vi "Start High-Speed Data Communication.vi"(0 "Device ID":i32, 1 "Max Buffer Size":u32, 7 "Ethernet Config":T1={"IP Address"=[192, 168, 0, 1], "Port No"=24692}, 9 "Start Req":T2={"High-Speed Comm Start Pos"=0, "Read Profile Cnt"=0, "High-Speed Receive Ratio"=16} {"High-Speed Receive Ratio" items=["LOWEST"=0, "LOW"=16, "MIDDLE"=17, "HIGH"=18, "HIGHEST"=32]; "High-Speed Comm Start Pos" items=["SEND COMPLETE POS", "OLDEST", "NEXT"]}, 11 "error in (no error)":errorcluster {"code" format="%.0x"}) -> (4 "Device ID out":i32, 15 "error out":errorcluster {"code" format="%.0x"})   [LabVIEW 2010, in "KEYENCE LJ-X8000A.lvlib"]
doc: "High-speed communication with the controller is established to start."
uses:
  KEYENCE LJ-X8000A.lvlib
  Clusters/Ethernet Config.ctl
  Clusters/High-Speed Comm Start Req.ctl
  Constants/High-Speed Comm Start Pos.ctl
  Constants/High-Speed Receive Ratio.ctl
panel:
  # "(c) 2019 KEYENCE CORPORATION.  ALL RIGHTS RESERVED."
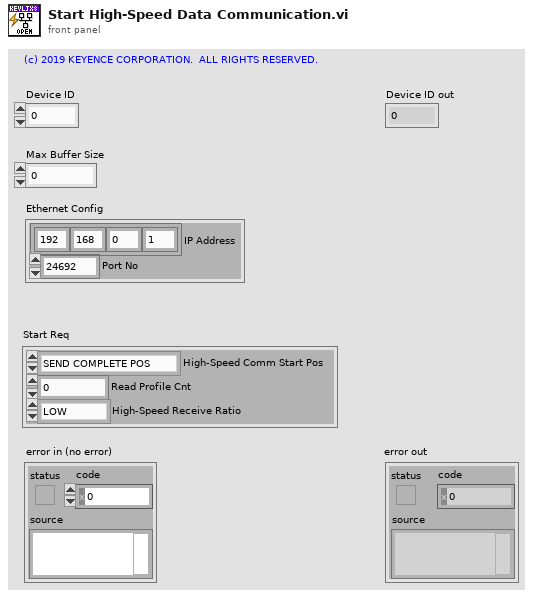
[diagram p1: front panel]
types:
  T1 = typedef "KEYENCE LJ-X8000A.lvlib/Ethernet Config.ctl" = cluster{"IP Address":u8[], "Port No":u16}
  T2 = typedef "KEYENCE LJ-X8000A.lvlib/High-Speed Comm Start Req.ctl" = cluster{"High-Speed Comm Start Pos":T3, "Read Profile Cnt":u32, "High-Speed Receive Ratio":T4}
  T3 = typedef "KEYENCE LJ-X8000A.lvlib/High-Speed Comm Start Pos.ctl" = u8
  T4 = typedef "KEYENCE LJ-X8000A.lvlib/High-Speed Receive Ratio.ctl" = u8
  T5 = cluster{"High-Speed Comm Start Pos":T3, "reserved":u8, "reserved":u8, "reserved":u8}
  T6 = cluster{"IP Address[0]":u8, "IP Address[1]":u8, "IP Address[2]":u8, "IP Address[3]":u8}
  T7 = cluster{"IP Address":cluster{"IP Address[0]":u8, "IP Address[1]":u8, "IP Address[2]":u8, "IP Address[3]":u8}, "Port No":u16, "reserved":u8, "reserved":u8}
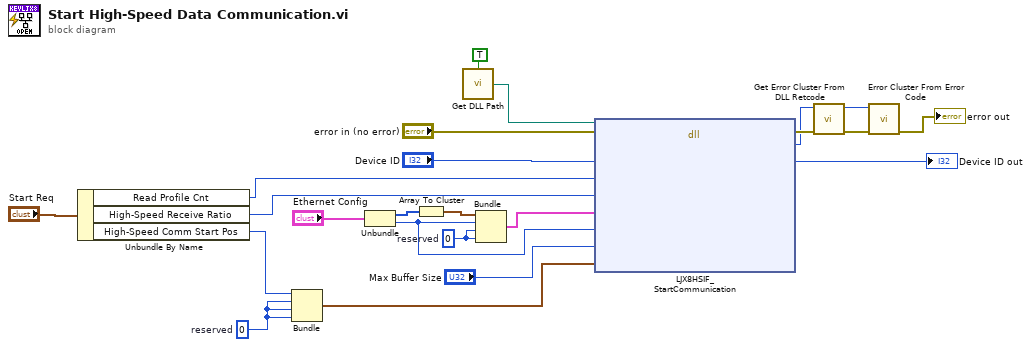
[diagram p0: block diagram]
diagram:
  w11 = u8 0  # reserved
  w16 = u8 0  # reserved
  n1 = Unbundle By Name("Start Req") -> ("Read Profile Cnt"=w19:u32, "High-Speed Receive Ratio"=w18:T4, "High-Speed Comm Start Pos"=w17:T3)
  n2 = Bundle("High-Speed Comm Start Pos"=w17, "reserved"=w16, "reserved"=w16, "reserved"=w16) -> (w15:T5)  [unwired: 1 in]
  n3 = Unbundle("Ethernet Config") -> ("IP Address"=w13:u8[], "Port No"=w9:u16)
  n4 = Array To Cluster(array=w13) -> (cluster=w12:T6)
  n5 = call "Get DLL Path.vi"("isWrapperDLL (False)"=TRUE) -> ("DLL Path"=w7:path)  [unwired: 2 in]
  n6 = Bundle("IP Address"=w12, "Port No"=w9, "reserved"=w11, "reserved"=w11) -> (w10:T7)  [unwired: 1 in]
  n7 = dll-call lib="C:/Program Files (x86)/National Instruments/LabVIEW 2018/instr.lib/KEYENCE LJ-X8000/LJX8_HighSpeedWrapper.*" fn="LJX8HSIF_StartCommunication"(path in=w7, error in="error in (no error)", "lDeviceId"="Device ID", "dwReqProfileCnt"=w19, "byReceiveRatio"=w18, "pEthernetConfig"=w10, "wHighSpeedPortNo"=w9, "dwMaxBufferSize"="Max Buffer Size", "pReq"=w15) -> (error out=w3:errorcluster, "lRetCode"=w1:i32, "lDeviceId"=→"Device ID out":i32)  [unwired: 7 in, 1 out]
  n8 = call "Get Error Cluster From DLL Retcode.vi"("error in (no error)"=w3, "DLL Return Code"=w1) -> ("error out"=w5:errorcluster, "VI Error Code"=w4:i32)  [unwired: 8 in]
  n9 = call <vilib>:"Error Cluster From Error Code.vi"("error in (no error)"=w5, "error code (0)"=w4) -> ("error out"=→"error out":errorcluster)  [unwired: 7 in]
